vi "create_vol_and_issue_date_job.vi"(8 "error in (no error)":errorcluster, 10 "job queue":refnum<queue>, 11 "job path":path) -> (0 "error out":errorcluster, 1 "job folder size":i32)   [LabVIEW 2024, in "Download_Manager.lvlib"]
uses:
  Download_Manager.lvlib
  typedefs/job--cluster.ctl
  typedefs/job_type--enum.ctl
  typedefs/volume_details--cluster.ctl
  <vilib>/addons/_JKI.lib/Serialization/JSON/JKI JSON Serialization.lvlib
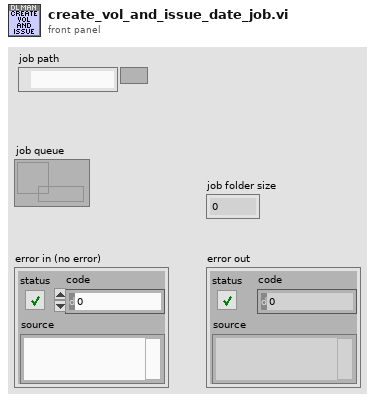
[diagram p1: front panel]
types:
  T1 = typedef "Download_Manager.lvlib/volume_details--cluster.ctl" = cluster{"id":i32, "issue_ids":i32[], "date_last_updated":timestamp, "Path":path}
  T2 = typedef "Download_Manager.lvlib/job_type--enum.ctl" = enum16{"check volume date", "check issues date", "download volume", "download isssue"}
  T3 = typedef "Download_Manager.lvlib/job--cluster.ctl" = cluster{"job type":T2, "job path":path, "id":i32, "url":string, "last updated":timestamp, "offset":i32, "original path":path}
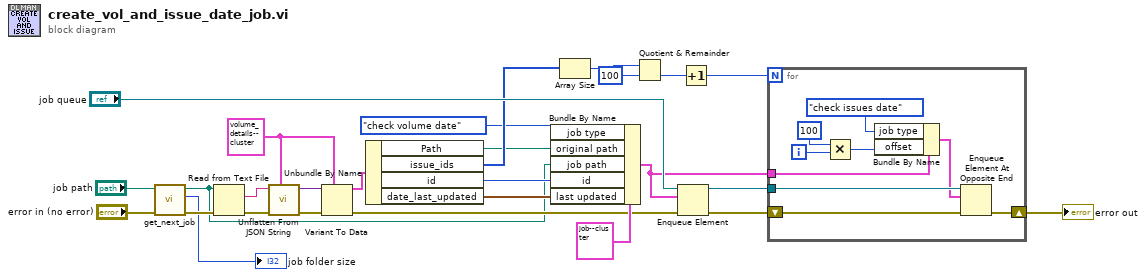
[diagram p0: block diagram]
diagram:
  w8 = T1 {"id"=0, "issue_ids"=[], "date_last_updated"=timestamp(0 s since 1904-01-01), "Path"=path ""} ("volume_details")
  n1 = call "get_next_job.vi"("error in (no error)"="error in (no error)", "cache path"="job path") -> ("error out"=w5:errorcluster, "remaining jobs"=→"job folder size":i32, "appended path"=w4:path)  [unwired: 7 in]
  n2 = Read from Text File(file (use dialog)=w4, error in=w5) -> (text=w21:string, error out=w20:errorcluster)  [unwired: 2 in, 2 out]
  n3 = call <vilib>:"Unflatten From JSON String.vi"("Type and Defaults"=w8, "error in"=w20, "JSON String"=w21) -> ("error out"=w22:errorcluster, "Variant"=w23:variant)  [unwired: 7 in]
  n4 = Variant To Data(error in=w22, type=w8, Variant=w23) -> (data=w24:T1, error out=w19:errorcluster)
  n5 = Unbundle By Name(w24) -> ("Path"=w2:path, "issue_ids"=w13:i32[], "id"=w26:i32, "date_last_updated"=w27:timestamp)
  n6 = Bundle By Name(cluster=T3 {"job type"=enum."check volume date", "job path"=path "", "id"=0, "url"="", "last updated"=timestamp(0 s since 1904-01-01), "offset"=0, "original path"=path ""} ("job"), "job type"=job_type--enum."check volume date", "original path"=w2, "job path"=w4, "id"=w26, "last updated"=w27) -> (w17:T3)
  n7 = Array Size(array=w13) -> (size(s)=w12:i32)
  n8 = Quotient & Remainder(x=w12, y=100) -> (floor(x/y)=w10:i32)  [unwired: 1 out]
  n9 = Enqueue Element(queue="job queue", element=w17, error in (no error)=w19) -> (queue out=w16:refnum<queue>, error out=w15:errorcluster)  [unwired: 1 in, 1 out]
  n10 = Increment(x=w10) -> (x+1=w9:i32)
  n11 = for {
    N: w9 -> [_]
    tunnel: w17 -> [w36]
    tunnel: w16 -> [w34]
    shift-right: [w31] -> w14
    shift-left: w15 -> [w33]
    i -> [w30]
    n12 = Multiply(x=100, y=w30) -> (x*y=w29:i32)
    n13 = Bundle By Name(cluster=w36, "job type"=job_type--enum."check issues date", "offset"=w29) -> (w32:T3)
    n14 = Enqueue Element At Opposite End(queue=w34, element=w32, error in (no error)=w33) -> (error out=w31:errorcluster)  [unwired: 1 in, 2 out]
  }
  "error out" <- w14
